vi "Read.vi"(8 "error in (no error)":errorcluster, 11 "Bronkhorst Settings in":T1) -> (0 "error out":errorcluster, 1 "Connection Error":bool, 2 "flow":dbl, 3 "Bronkhorst Settings out":T1)   [LabVIEW 2018, in "Bronkhorst M14 Flow Meter.lvlib"]
uses:
  Bronkhorst M14 Flow Meter.lvlib
  Settings Cluster.ctl
  <vilib>/regexp/Match Regular Expression.xnode
  <vilib>/ptbypt/NI_PtbyPt.lvlib
panel:
  out "submatch 1":string
  out "Waveform Chart":u32(graph)
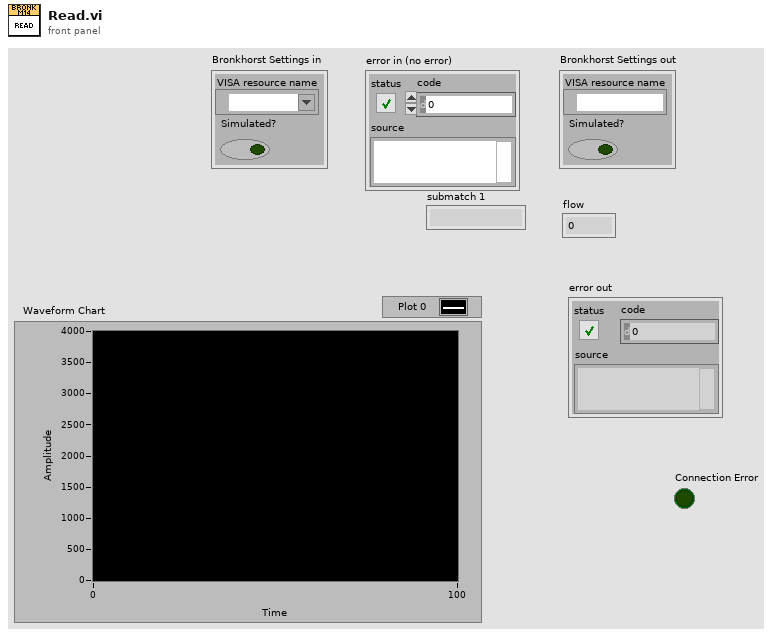
[diagram p1: front panel]
types:
  T1 = typedef "Bronkhorst M14 Flow Meter.lvlib/Settings Cluster.ctl" = cluster{"VISA resource name":refnum<visa-resource-name>, "Simulated?":bool}
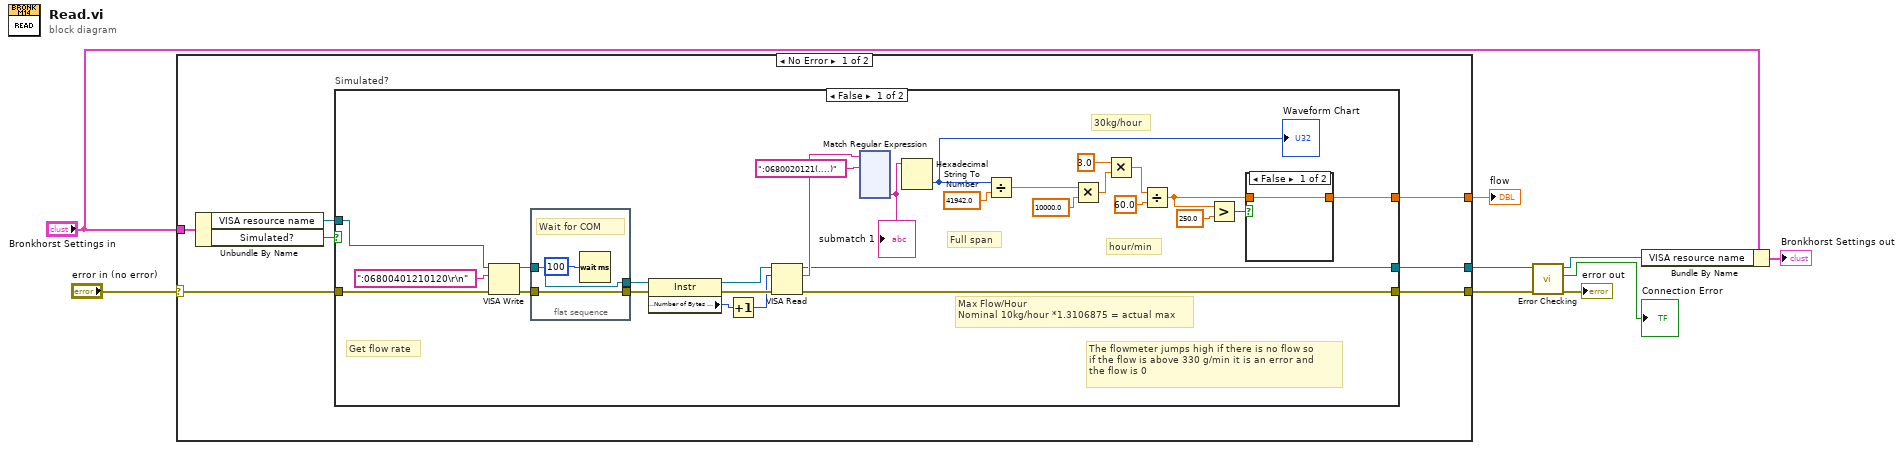
[diagram p0: block diagram]
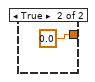
[diagram p2: hidden frame]
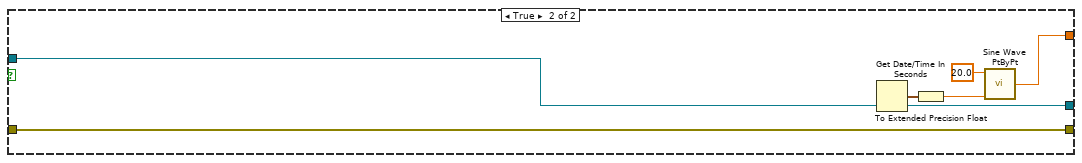
[diagram p3: hidden frame]
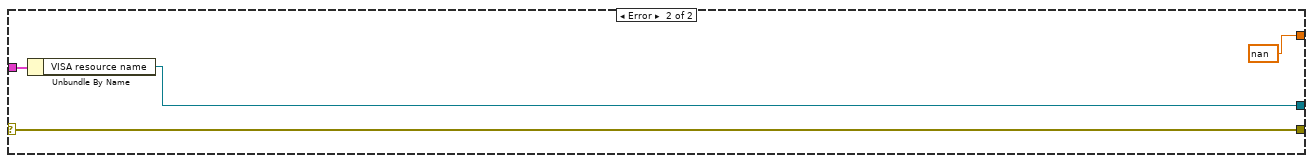
[diagram p4: hidden frame]
diagram:
  n1 = case shown="No Error" "error in (no error)" {
    selector: "error in (no error)" -> [w15 w175]
    tunnel: [w14 w175] -> w3
    tunnel: "Bronkhorst Settings in" -> [w12 w173]
    tunnel: [w13 nan ("sine wave")] -> w9
    tunnel: [w10 w172] -> w5
    frame No Error {
      n2 = Unbundle By Name(w12) -> ("VISA resource name"=w11:refnum<visa-resource-name>, "Simulated?"=w16:bool)
      n3 = case "Simulated?" shown="False" w16 {
        tunnel: [w21 w171] -> w14
        tunnel: w15 -> [w26 w171]
        tunnel: [w29 w167] -> w13
        tunnel: [w22 w166] -> w10
        tunnel: w11 -> [w27 w166]
        frame False {
          # "30kg/hour"
          # "hour/min"
          # "Max Flow/Hour\nNominal 10kg/hour *1.3106875 = actual max"
          # "Get flow rate"
          # "The flowmeter jumps high if there is no flow so \nif the flow is above 330 g/min it is an error and \nthe flow is 0"
          # "Full span"
          n4 = VISA Write(VISA resource name=w27, write buffer=":06800401210120\r\n" ("Command"), error in (no error)=w26) -> (VISA resource name out=w41:refnum<visa-resource-name>, error out=w39:errorcluster)  [unwired: 1 out]
          n5 = flat-sequence {
            tunnel: [w165] -> w40
            tunnel: w41 -> [w165]
            tunnel: [w164] -> w38
            tunnel: w39 -> [w164]
            frame #0 {
              # "Wait for COM"
              n6 = Wait (ms)(milliseconds to wait=u32 100) -> ()  [unwired: 1 out]
            }
          }
          n7 = property class="Instr"(reference=w40, error in=w38) -> (reference out=w43:refnum<visa-resource-name>, error out=w42:errorcluster, "Serial Settings:Number of Bytes at Serial Port"=w24:u32)
          n8 = Increment(x=w24) -> (x+1=w23:u32)
          n9 = VISA Read(VISA resource name=w43, byte count=w23, error in (no error)=w42) -> (VISA resource name out=w22:refnum<visa-resource-name>, read buffer=w25:string, error out=w21:errorcluster)  [unwired: 1 out]
          n10 = xnode "Match Regular Expression"("input string"=w25, "regular expression"=":0680020121(....)" ("Regular Expression for Extracting Weight")) -> ("submatch 1"=w20:string)  [unwired: 4 in, 5 out]
          "submatch 1" <- w20
          n11 = Hexadecimal String To Number(string=w20) -> (number=w28:u32)  [unwired: 2 in, 1 out]
          "Waveform Chart" <- w28
          n12 = Divide(x=w28, y=41942.0) -> (x/y=w32:dbl)
          n13 = Multiply(x=w32, y=10000.0) -> (x*y=w19:dbl)
          n14 = Multiply(x=3.0, y=w19) -> (x*y=w18:dbl)
          n15 = Divide(x=w18, y=60.0) -> (x/y=w30:dbl)
          n16 = Greater?(x=w30, y=250.0) -> (0:w31:bool)
          n17 = case shown="False" w31 {
            tunnel: [w45 0.0] -> w29
            tunnel: w30 -> [w45 _]
            frame False {
            }
            frame True {
            }
          }
        }
        frame True {
          n18 = Get Date/Time In Seconds() -> (seconds since 1Jan1904=w170:timestamp)
          n19 = To Extended Precision Float(1:w170) -> (0:w169:ext)
          n20 = call <vilib>:"Sine Wave PtByPt.vi"("time"=w169, "amplitude"=20.0) -> ("sine wave"=w167:dbl)  [unwired: 2 in]
        }
      }
    }
    frame Error {
      n21 = Unbundle By Name(w173) -> ("VISA resource name"=w172:refnum<visa-resource-name>)
    }
  }
  "flow" <- w9
  n22 = call "Error Checking.vi"("error in (no error)"=w3, "VISA resource name"=w5) -> ("error out"=→"error out":errorcluster, "Connection Error"=→"Connection Error":bool, "VISA resource name"=w4:refnum<visa-resource-name>)  [unwired: 7 in]
  n23 = Bundle By Name(cluster="Bronkhorst Settings in", "VISA resource name"=w4) -> (→"Bronkhorst Settings out":T1)
